vi "Test ARGB Data to Pixel Data.vi"(8 "error in (no error)":errorcluster, 11 "Test Case In":refnum<class "01_Image.lvclass">) -> (0 "error out":errorcluster, 3 "Test Case Out":refnum<class "01_Image.lvclass">)   [LabVIEW 2020, in "test.lvlib" / "01_Image.lvclass"]
uses:
  01_Image.lvclass
  C:/Program Files (x86)/National Instruments/LabVIEW 2026/vi.lib/Astemes/LUnit/Test Case.lvclass
  common/Image Size (Integer).ctl
  <vilib>/Astemes/LUnit/Test Case.lvclass/Test Case.ctl
  4993e8ee-a06a-463a-9684-69129f64d5ce.vi
  eb111072-ef64-4670-bf69-e7e9452429d1.vi
  image/New Image.vi
  image/New Image (ARGB Preallocated).vi
  image/Copy Array to Image.vi
  image/Copy Array to Image (ARGB).vi
  <vilib>/Astemes/LUnit/Core/LUnit Test Case/Private/Append Pass Result.vi
  <vilib>/Astemes/LUnit/Core/LUnit Test Case/Private/Append Fail Result.vi
  4993e8ee-a06a-463a-9684-69129f64d5ce.vi/9c5d11cd-9439-4240-a1ee-d9baace9c924.vi
  eb111072-ef64-4670-bf69-e7e9452429d1.vi/9c5d11cd-9439-4240-a1ee-d9baace9c924.vi
  image/New Image (ARGB Preallocated).vi/3321fa97-f432-4e1e-8db9-a0df79aed21b.vi
  image/ARGB Colour to U32 Pixel Value.vi
  <vilib>/Astemes/LUnit/Core/LUnit Test Case/Private/Run In UI.vi
  <vilib>/Utility/error.llb/Clear Errors.vi
  <vilib>/Utility/error.llb/Error Cluster From Error Code.vi
  <vilib>/picture/pixmap.llb/Flatten Pixmap.vi
  image/image.lvlib
  common/common.lvlib
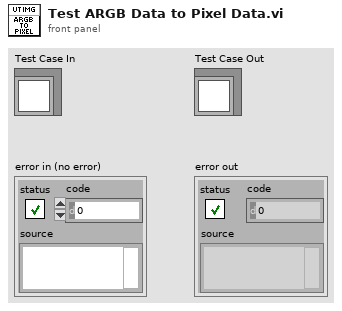
[diagram p1: front panel]
types:
  T1 = typedef "common.lvlib/Image Size (Integer).ctl" = cluster{"Width":u16, "Height":u16}
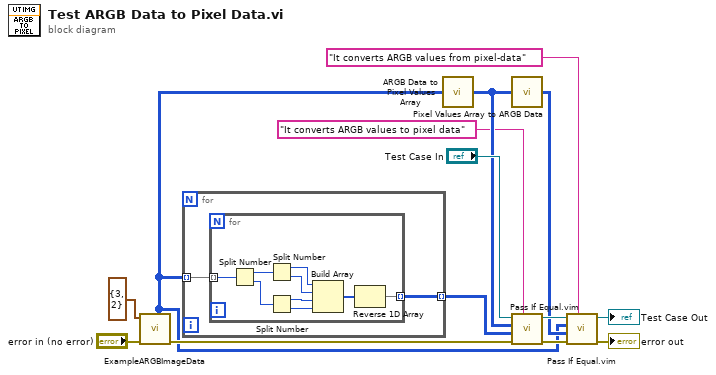
[diagram p0: block diagram]
diagram:
  n1 = call "ExampleARGBImageData.vi"("error in (no error)"="error in (no error)", "Image Size"=T1 {"Width"=3, "Height"=2}) -> ("error out"=w3:errorcluster, "ARGB Array Data"=w1:u32[][])  [unwired: 6 in, 2 out]
  n2 = for {
    tunnel: w1 -> [w16] mode=indexing
    tunnel: [w15] -> w13 mode=indexing
    n3 = for {
      tunnel: w16 -> [w25] mode=indexing
      tunnel: [w17] -> w15 mode=indexing
      n4 = Split Number(x=w25) -> (hi(x)=w24:u16, lo(x)=w23:u16)
      n5 = Split Number(x=w24) -> (hi(x)=w21:u8, lo(x)=w20:u8)
      n6 = Split Number(x=w23) -> (hi(x)=w19:u8, lo(x)=w18:u8)
      n7 = Build Array(w21, w20, w19, w18) -> (w22:u8[])
      n8 = Reverse 1D Array(array=w22) -> (reversed array=w17:u8[])
    }
  }
  n9 = call "ARGB Data to Pixel Values Array.vi"("ARGB Data"=w1) -> ("Pixel Values"=w12:u8[][][])
  n10 = call "Pixel Values Array to ARGB Data.vi"("Pixel Values"=w12) -> ("ARGB Data"=w6:u32[][])
  n11 = call "Pass If Equal.vim"("Description"="It converts ARGB values to pixel data", "error in (no error)"=w3, "Actual"=w13, "Expected"=w12, "LUnit Test Case In"="Test Case In") -> ("error out"=w10:errorcluster, "LUnit Test Case Out"=w9:refnum<class "01_Image.lvclass">)  [unwired: 5 in]
  n12 = call "Pass If Equal.vim"("Description"="It converts ARGB values from pixel-data", "error in (no error)"=w10, "Actual"=w6, "Expected"=w1, "LUnit Test Case In"=w9) -> ("error out"=→"error out":errorcluster, "LUnit Test Case Out"=→"Test Case Out":refnum<class "01_Image.lvclass">)  [unwired: 5 in]
